vi "CoboltLaser_OperatingHoursGet.vi"(0 "ComPort":refnum<visa-resource-name>, 3 "CheckResponse":bool=TRUE, 7 "error in (no error)":errorcluster) -> (20 "ComPortOut":refnum<visa-resource-name>, 21 "OperatingHours":dbl, 27 "error out":errorcluster)   [LabVIEW 2012, in "Cobolt.lvclass"]
doc: "Use this template to build a VI to use as a subVI."
uses:
  Template/Cobolt.lvclass
panel:
  out "ResponseOK":bool
  out "Response":string
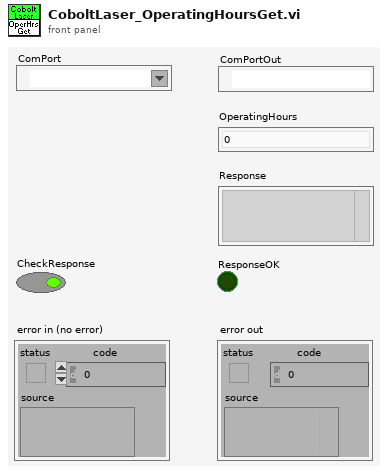
[diagram p1: front panel]
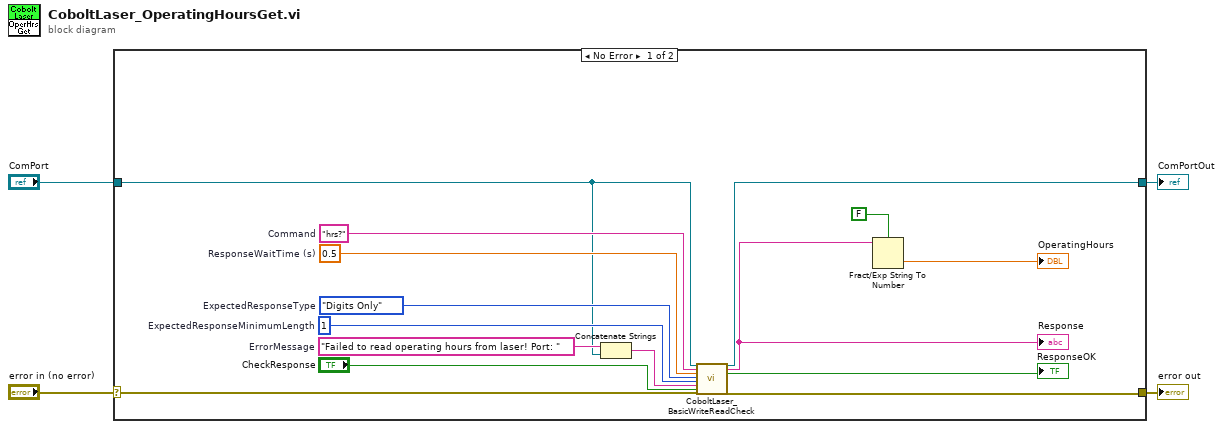
[diagram p0: block diagram]
diagram:
  n1 = case shown="No Error" "error in (no error)" {
    selector: "error in (no error)" -> [w19 w21]
    tunnel: [w18 w21] -> w3
    tunnel: "ComPort" -> [w7 w20]
    tunnel: [w6 w20] -> w1
    frame No Error {
      w14 = 1  # ExpectedResponseMinimumLength
      w15 = enum16{"Any", "Digits Only", "Non-Digits Only"}."Digits Only"  # ExpectedResponseType
      w17 = 0.5  # ResponseWaitTime (s)
      w11 = "Failed to read operating hours from laser! Port: "  # ErrorMessage
      w16 = "hrs?"  # Command
      n2 = Concatenate Strings(w11, w7) -> (w10:string)
      n3 = call "CoboltLaser_BasicWriteReadCheck.vi"("ComPort"=w7, "Command"=w16, "ResponseWaitTime (s)"=w17, "ExpectedResponseType"=w15, "ExpectedResponseMinimumLength"=w14, "ErrorMessage"=w10, "CheckResponse"="CheckResponse", "error in (no error)"=w19) -> ("ComPortOut"=w6:refnum<visa-resource-name>, "Response"=w9:string, "ResponseOK"=→"ResponseOK":bool, "error out"=w18:errorcluster)  [unwired: 16 in]
      "Response" <- w9
      n4 = Fract/Exp String To Number(use system decimal point (T)=FALSE, string=w9) -> (number=→"OperatingHours":dbl)  [unwired: 2 in, 1 out]
    }
    frame Error {
    }
  }
  "error out" <- w3
  "ComPortOut" <- w1
